vi "ShiftRegister-Generic.vi"() -> ()   [LabVIEW 2020]
doc: "Use this template to create an application that executes repeatedly until you click the Stop button. This template polls the state of the Stop button and does not use events. Use the Top-Level Application template (not available in the Base package) to create a single-loop application with event handling."
panel:
  in  "Write Data":dbl
  out "Data Read":dbl
  in  "Operate":T1(ring)
  out "error out":errorcluster
  in  "error in":errorcluster
  in  "stop":bool
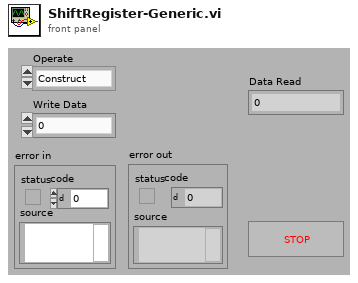
[diagram p1: front panel]
types:
  T1 = enum16{"Construct", "Initialize", "Read", "Write", "DeConstruct"}
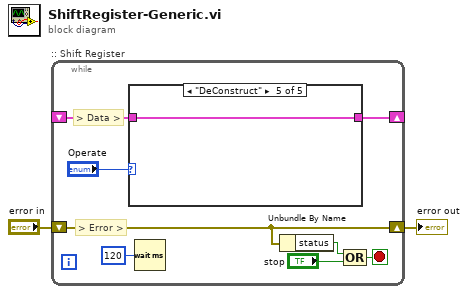
[diagram p0: block diagram]
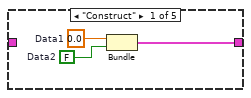
[diagram p2: hidden frame]
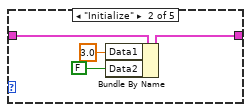
[diagram p3: hidden frame]
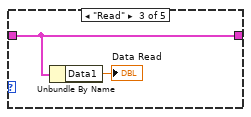
[diagram p4: hidden frame]
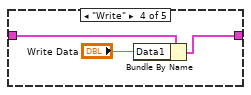
[diagram p5: hidden frame]
diagram:
  n1 = while ":: Shift Register" {
    shift-right: [w7] -> _
    shift-left: _ -> [w8]
    shift-right: [w10] -> w1
    shift-left: "error in" -> [w10]
    stop <- w4 stop-if-true
    # "> Data >"
    # "> Error >"
    n2 = case shown="\"DeConstruct\"" "Operate" {
      tunnel: w8 -> [_ w17 w19 w21 w23]
      tunnel: [w12 w16 w19 w20 w23] -> w7
      frame "Construct" {
        w11 = FALSE  # Data2
        w13 = 0.0  # Data1
        n3 = Bundle("Data1"=w13, "Data2"=w11) -> (w12:cluster{"Data1":dbl, "Data2":bool})  [unwired: 1 in]
      }
      frame "Initialize" {
        n4 = Bundle By Name(cluster=w17, "Data1"=3.0, "Data2"=FALSE) -> (w16:cluster{"Data1":dbl, "Data2":bool})
      }
      frame "Read" {
        n5 = Unbundle By Name(w19) -> ("Data1"=→"Data Read":dbl)
      }
      frame "Write" {
        n6 = Bundle By Name(cluster=w21, "Data1"="Write Data") -> (w20:cluster{"Data1":dbl, "Data2":bool})
      }
      frame "DeConstruct" {
      }
    }
    n7 = Wait (ms)(milliseconds to wait=u32 120) -> ()  [unwired: 1 out]
    n8 = Unbundle By Name(w10) -> ("status"=w6:bool)
    n9 = Compound Arithmetic op=OR(w6, "stop") -> (w4:bool)
  }
  "error out" <- w1
